vi "Pos Processamento.vi"(1 "task/channels in":refnum<k21>="ADQUIRE", 2 "file path":path) -> ()   [LabVIEW 2019]
uses:
  <vilib>/Utility/file.llb/Read Delimited Spreadsheet (string).vi
  <vilib>/Utility/file.llb/Write Delimited Spreadsheet (string).vi
  <vilib>/Utility/file.llb/Write Delimited Spreadsheet (DBL).vi
panel:
  in  "indexAux":dbl
  out "max":dbl[](array[numeric])
  out "min":dbl[](array[numeric])
  out "output":dbl[][](array[numeric])
  out "output_mA":dbl[][](array[numeric])
  # "indexAux armazena qual a posição\ndeve ser lida dos valores de máximo e mínimo"
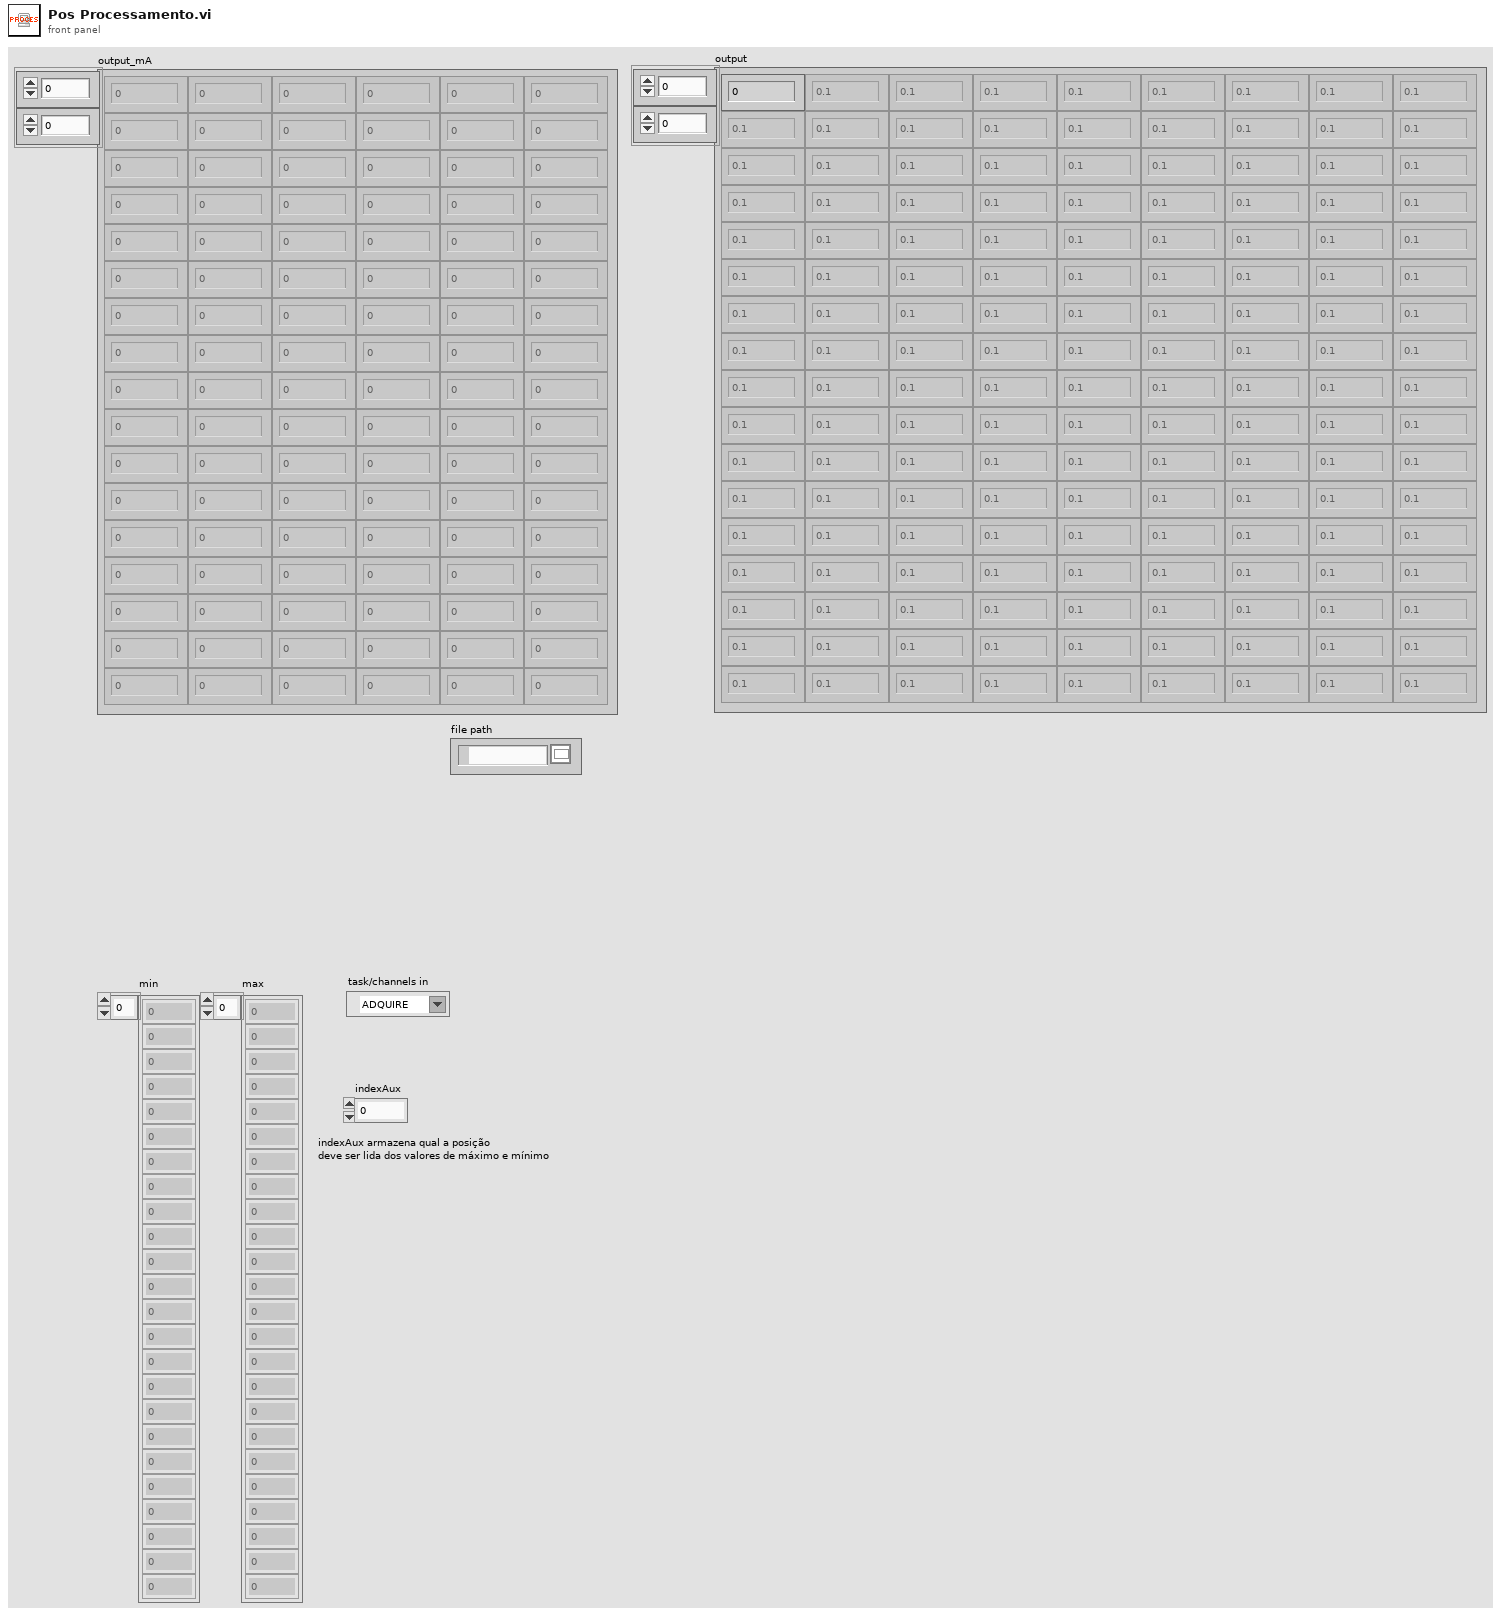
[diagram p1: front panel]
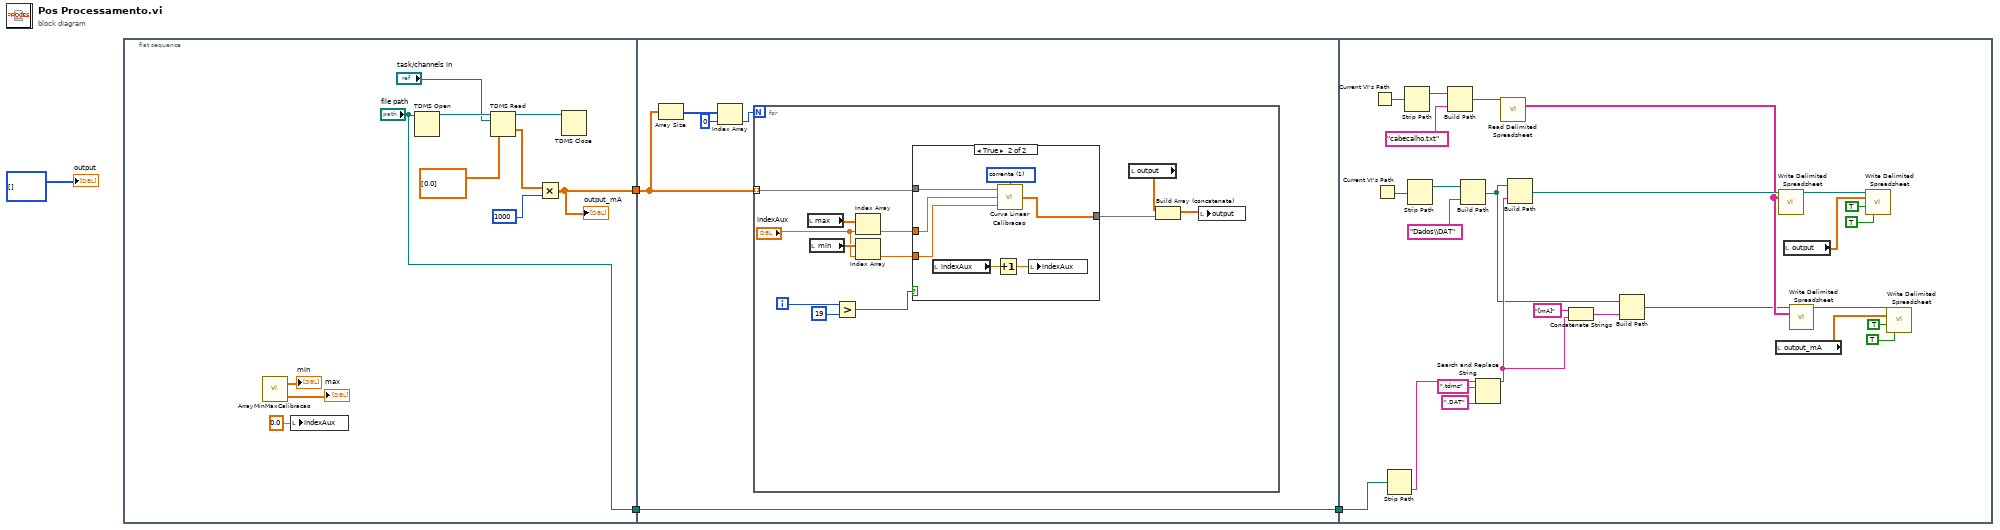
[diagram p0: block diagram]
diagram:
  n1 = flat-sequence {
    tunnel: [w12] -> w4
    tunnel: ["file path"] -> w3
    tunnel: w4 -> [w20]
    tunnel: w3 -> [w16]
    tunnel: [w16] -> w1
    tunnel: w1 -> [w62]
    frame #0 {
      n2 = call "ArrayMinMaxCalibracao.vi"() -> ("max"=→"max":dbl[], "min"=→"min":dbl[])  [unwired: 2 in]
      n3 = local write "indexAux"(0.0 ("indexAux")) -> ()
      n4 = TDMS Open(11:"file path") -> (3:w15:refnum<k34>)  [unwired: 6 in, 1 out]
      n5 = TDMS Read(0:w15, 5:"task/channels in", 12:dbl[][] [[0.0]] ("data")) -> (4:w14:refnum<k34>, 10:w11:dbl[][])  [unwired: 5 in, 4 out]
      n6 = Multiply(x=w11, y=1000 ("Numeric")) -> (x*y=w12:dbl[][])
      "output_mA" <- w12
      n7 = TDMS Close(11:w14) -> ()  [unwired: 1 in, 2 out]
    }
    frame #1 {
      n8 = Array Size(array=w20) -> (size(s)=w19:i32[])
      n9 = Index Array(array=w19, index=0) -> (element=w17:i32)
      n10 = for {
        N: w17 -> [_]
        tunnel: w20 -> [w32] mode=indexing
        i -> [w23]
        n11 = local read "max"() -> (w28:dbl[])
        n12 = local read "min"() -> (w27:dbl[])
        n13 = Greater?(x=w23, y=19) -> (0:w22:bool)
        n14 = Index Array(array=w28, index="indexAux") -> (element=w26:dbl)
        n15 = Index Array(array=w27, index="indexAux") -> (element=w25:dbl)
        n16 = case shown="True" w22 {
          tunnel: w32 -> [w33 w40]
          tunnel: [w33 w39] -> w29
          tunnel: w26 -> [_ w37]
          tunnel: w25 -> [_ w36]
          frame False {
          }
          frame True {
            w38 = u16 1 items=["tensao", "corrente"] ("input type")
            n17 = local read "indexAux"() -> (w35:dbl)
            n18 = Increment(x=w35) -> (x+1=w34:dbl)
            n19 = call "Curva Linear Calibracao.vi"("input type"=w38, "MIN"=w36, "MAX"=w37, "input"=w40) -> ("output"=w39:dbl[])
            n20 = local write "indexAux"(w34) -> ()
          }
        }
        n21 = local read "output"() -> (w30:dbl[][])
        n22 = Build Array (concatenate)(w30, w29) -> (w31:dbl[][])
        n23 = local write "output"(w31) -> ()
      }
    }
    frame #2 {
      n24 = Current VI's Path() -> (path=w66:path)
      n25 = Current VI's Path() -> (path=w61:path)
      n26 = Strip Path(path=w62) -> (name=w56:string)  [unwired: 1 out]
      n27 = Strip Path(path=w66) -> (stripped path=w65:path)  [unwired: 1 out]
      n28 = Strip Path(path=w61) -> (stripped path=w59:path)  [unwired: 1 out]
      n29 = Build Path(base path=w65, name or relative path="cabecalho.txt") -> (appended path=w63:path)
      n30 = Build Path(base path=w59, name or relative path="Dados\\DAT") -> (appended path=w42:path)
      n31 = Search and Replace String(input string=w56, search string=".tdms", replace string=".DAT" ("replace string (\"\")")) -> (result string=w44:string)  [unwired: 5 in, 3 out]
      n32 = call-poly <vilib>:"Read Delimited Spreadsheet.vi"("file path (dialog if empty)"=w63) -> ("all rows"=w46:string[][])  [unwired: 9 in, 5 out]
      n33 = Build Path(base path=w42, name or relative path=w44) -> (appended path=w55:path)
      n34 = Concatenate Strings("[mA]" ("string"), w44) -> (w43:string)
      n35 = Build Path(base path=w42, name or relative path=w43) -> (appended path=w41:path)
      n36 = local read "output_mA"() -> (w48:dbl[][])
      n37 = call-poly <vilib>:"Write Delimited Spreadsheet.vi"("file path (dialog if empty)"=w55, "2D data"=w46) -> ("new file path (Not A Path if cancelled)"=w54:path)  [unwired: 12 in, 1 out]
      n38 = local read "output"() -> (w53:dbl[][])
      n39 = call-poly <vilib>:"Write Delimited Spreadsheet.vi"("file path (dialog if empty)"=w41, "2D data"=w46) -> ("new file path (Not A Path if cancelled)"=w47:path)  [unwired: 12 in, 1 out]
      n40 = call-poly <vilib>:"Write Delimited Spreadsheet.vi"("file path (dialog if empty)"=w54, "2D data"=w53, "append to file? (new file:F)"=TRUE, "transpose? (no:F)"=TRUE) -> ()  [unwired: 10 in, 2 out]
      n41 = call-poly <vilib>:"Write Delimited Spreadsheet.vi"("file path (dialog if empty)"=w47, "2D data"=w48, "append to file? (new file:F)"=TRUE, "transpose? (no:F)"=TRUE) -> ()  [unwired: 10 in, 2 out]
    }
  }
  "output" <- i32[][] [] ("data")
